vi "Get Axis Name.vi"(8 "error in (no error)":errorcluster, 11 "SIM Motion Controller in":refnum<class "Fine SIM Motion Controller.lvclass">) -> (0 "error out":errorcluster, 2 "Axis Name":string, 3 "SIM Motion Controller out":refnum<class "Fine SIM Motion Controller.lvclass">)   [LabVIEW 2022 SP3, in "Fine SIM Motion Controller.lvclass"]
uses:
  Fine SIM Motion Controller.lvclass
  Fine SIM Motion Controller.lvclass/Fine SIM Motion Controller.ctl
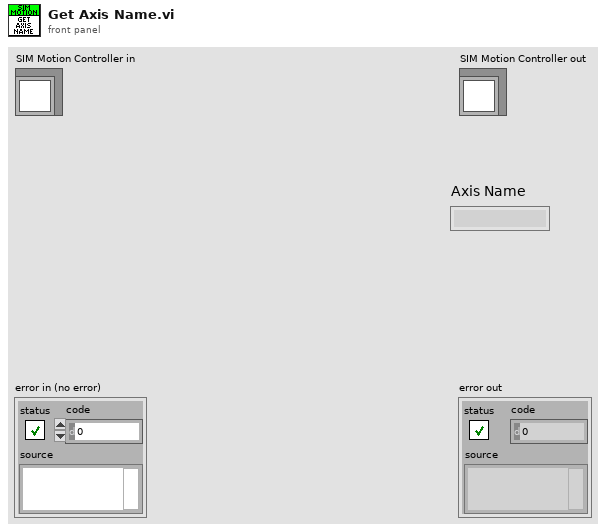
[diagram p1: front panel]
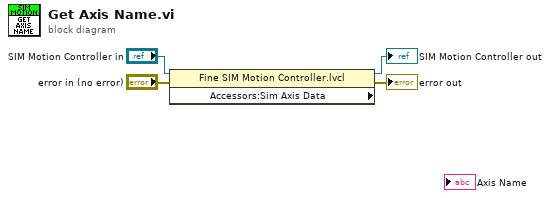
[diagram p0: block diagram]
diagram:
  n1 = property class="Fine SIM Motion Controller.lvcl" props=["Accessors:Sim Axis Data"](reference="SIM Motion Controller in", error in="error in (no error)") -> (reference out=→"SIM Motion Controller out":refnum<class "Fine SIM Motion Controller.lvclass">, error out=→"error out":errorcluster)  [unwired: 1 out]
